vi "TimeDriven.vi"() -> ()   [LabVIEW 2018]
uses:
  FGV/FGV_mods.ctl
  AE/timeMark_data.ctl
  <vilib>/Analysis/NI_AALPro.lvlib
panel:
  out "b":dbl
  out "a":dbl
  out "Histórico":cluster{dbl[], dbl[]}[](graph)
  in  "file":path caption="Arquivo"
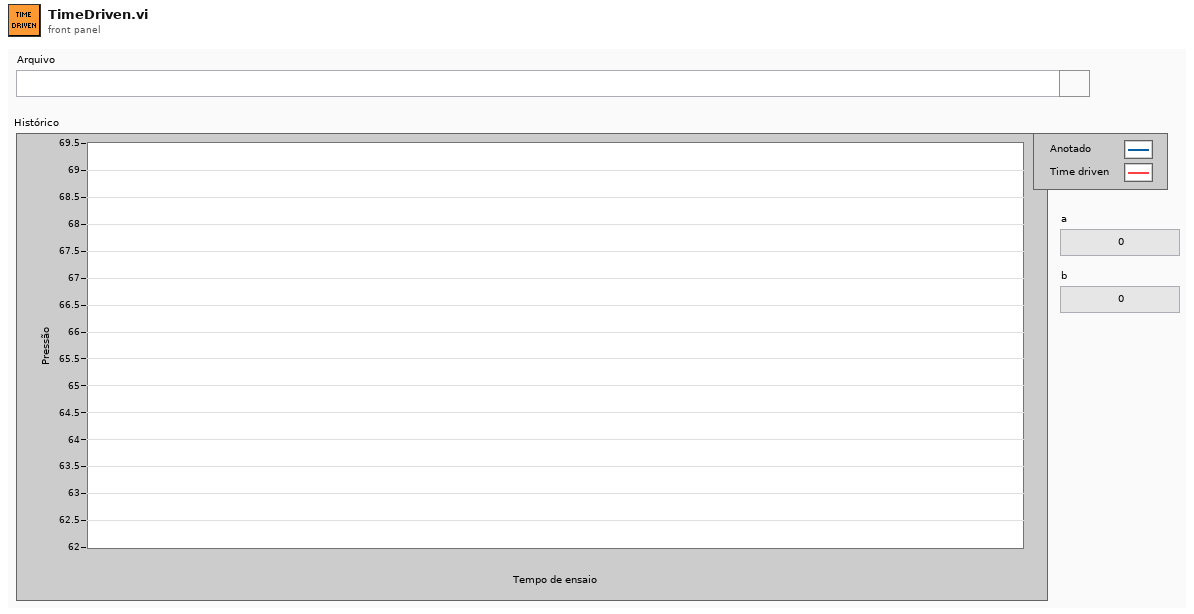
[diagram p1: front panel]
types:
  T1 = typedef "timeMark_data.ctl" = cluster{"time":dbl, "message":string}
  T2 = typedef "FGV_mods.ctl" = enum16{"Init", "get_config", "get_hits", "get_timeDriven", "get_timeMarks", "set_file", "open_file", "get_startTime", "close"}
  T3 = typedef "timeDriven_data.ctl" = cluster{"time":dbl, "parametrics":i16[]}
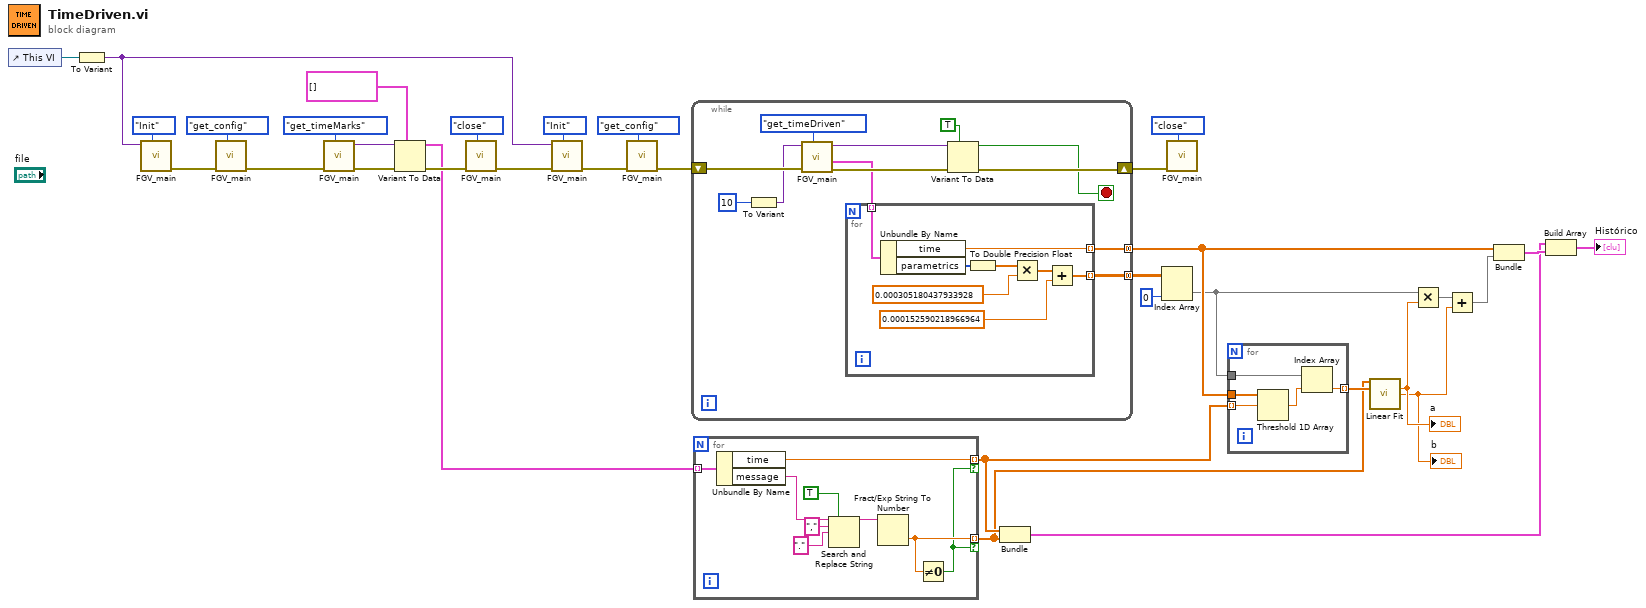
[diagram p0: block diagram]
diagram:
  n1 = control-ref of="This VI"() -> (w29:refnum<vi>)
  n2 = To Variant(anything=w29) -> (Variant=w18:variant)
  n3 = call "FGV_main.vi"("FGV_mods"=FGV_mods."Init", "DataIn"=w18) -> ("Error Out"=w32:errorcluster)  [unwired: 6 in, 3 out]
  n4 = call "FGV_main.vi"("FGV_mods"=FGV_mods."get_config", "Error In"=w32) -> ("Error Out"=w25:errorcluster)  [unwired: 6 in, 3 out]
  n5 = call "FGV_main.vi"("FGV_mods"=FGV_mods."get_timeMarks", "Error In"=w25) -> ("Error Out"=w17:errorcluster, "DataOut"=w16:variant)  [unwired: 6 in, 2 out]
  n6 = Variant To Data(error in=w17, type=T1[] [] ("data"), Variant=w16) -> (data=w13:T1[], error out=w14:errorcluster)
  n7 = call "FGV_main.vi"("FGV_mods"=FGV_mods."close", "Error In"=w14) -> ("Error Out"=w20:errorcluster)  [unwired: 6 in, 3 out]
  n8 = call "FGV_main.vi"("FGV_mods"=FGV_mods."Init", "Error In"=w20, "DataIn"=w18) -> ("Error Out"=w23:errorcluster)  [unwired: 5 in, 3 out]
  n9 = call "FGV_main.vi"("FGV_mods"=FGV_mods."get_config", "Error In"=w23) -> ("Error Out"=w19:errorcluster)  [unwired: 6 in, 3 out]
  n10 = while {
    shift-right: [w39] -> w30
    shift-left: w19 -> [w45]
    tunnel: [w36] -> w28 mode=concatenating
    tunnel: [w35] -> w8 mode=concatenating
    stop <- w38 stop-if-true
    n11 = To Variant(anything=10) -> (Variant=w43:variant)
    n12 = call "FGV_main.vi"("FGV_mods"=FGV_mods."get_timeDriven", "Error In"=w45, "DataIn"=w43) -> ("Error Out"=w40:errorcluster, "timeDriven"=w37:T3[], "DataOut"=w42:variant)  [unwired: 5 in, 1 out]
    n13 = for {
      tunnel: w37 -> [w54] mode=indexing
      tunnel: [w48] -> w36 mode=indexing
      tunnel: [w47] -> w35 mode=indexing
      n14 = Unbundle By Name(w54) -> ("time"=w47:dbl, "parametrics"=w53:i16[])
      n15 = To Double Precision Float(number=w53) -> (double precision float=w52:dbl[])
      n16 = Multiply(x=w52, y=0.000305180437933928) -> (x*y=w50:dbl[])
      n17 = Add(x=w50, y=0.000152590218966964) -> (x+y=w48:dbl[])
    }
    n18 = Variant To Data(error in=w40, type=TRUE, Variant=w42) -> (data=w38:bool, error out=w39:errorcluster)
  }
  n19 = for {
    tunnel: w13 -> [w63] mode=indexing
    tunnel: [w57] -> w9 mode=indexing if=w55
    tunnel: [w56] -> w6 mode=indexing if=w55
    n20 = Unbundle By Name(w63) -> ("time"=w57:dbl, "message"=w62:string)
    n21 = Search and Replace String(replace all?=TRUE ("replace all? (F)"), input string=w62, search string=",", replace string="." ("search string")) -> (result string=w58:string)  [unwired: 4 in, 3 out]
    n22 = Fract/Exp String To Number(string=w58) -> (number=w56:dbl)  [unwired: 3 in, 1 out]
    n23 = Not Equal To 0?(x=w56) -> (x != 0?=w55:bool)
  }
  n24 = Bundle(w9, w6) -> (w11:cluster{dbl[], dbl[]})  [unwired: 1 in]
  n25 = Index Array(array=w28, index (col)=0 ("disabled index (col)")) -> (element=w5:dbl[])  [unwired: 1 in]
  n26 = call "FGV_main.vi"("FGV_mods"=FGV_mods."close", "Error In"=w30) -> ()  [unwired: 6 in, 4 out]
  n27 = for {
    tunnel: w9 -> [w67] mode=indexing
    tunnel: w8 -> [w68]
    tunnel: w5 -> [w66]
    tunnel: [w64] -> w7 mode=indexing
    n28 = Threshold 1D Array(2:w67, 3:w68) -> (0:w65:dbl)  [unwired: 1 in]
    n29 = Index Array(array=w66, index=w65) -> (element=w64:dbl)
  }
  n30 = call <vilib>:"Linear Fit.vi"("Y"=w6, "X"=w7) -> ("slope"=w2:dbl, "intercept"=w1:dbl)  [unwired: 9 in, 3 out]
  "a" <- w2
  "b" <- w1
  n31 = Multiply(x=w5, y=w2) -> (x*y=w4:dbl[])
  n32 = Add(x=w4, y=w1) -> (x+y=w3:dbl[])
  n33 = Bundle(w8, w3) -> (w12:cluster{dbl[], dbl[]})  [unwired: 1 in]
  n34 = Build Array(w11, w12) -> (→"Histórico":cluster{dbl[], dbl[]}[])
